vi "HDF5 Index.vi"(8 "error in (no error)":errorcluster, 11 "Mapping Type":enum16{"Dataset", "Variables"}(ring)=enum."Variables") -> (0 "error out":errorcluster, 3 "Mapping out":i32[](array[numeric]))   [LabVIEW 2011]
uses:
  User Interface VIs.lvlib
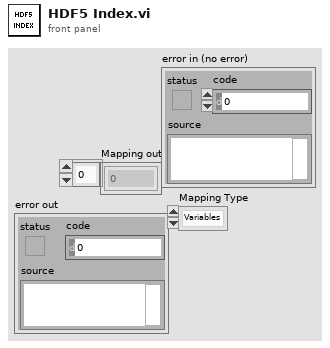
[diagram p1: front panel]
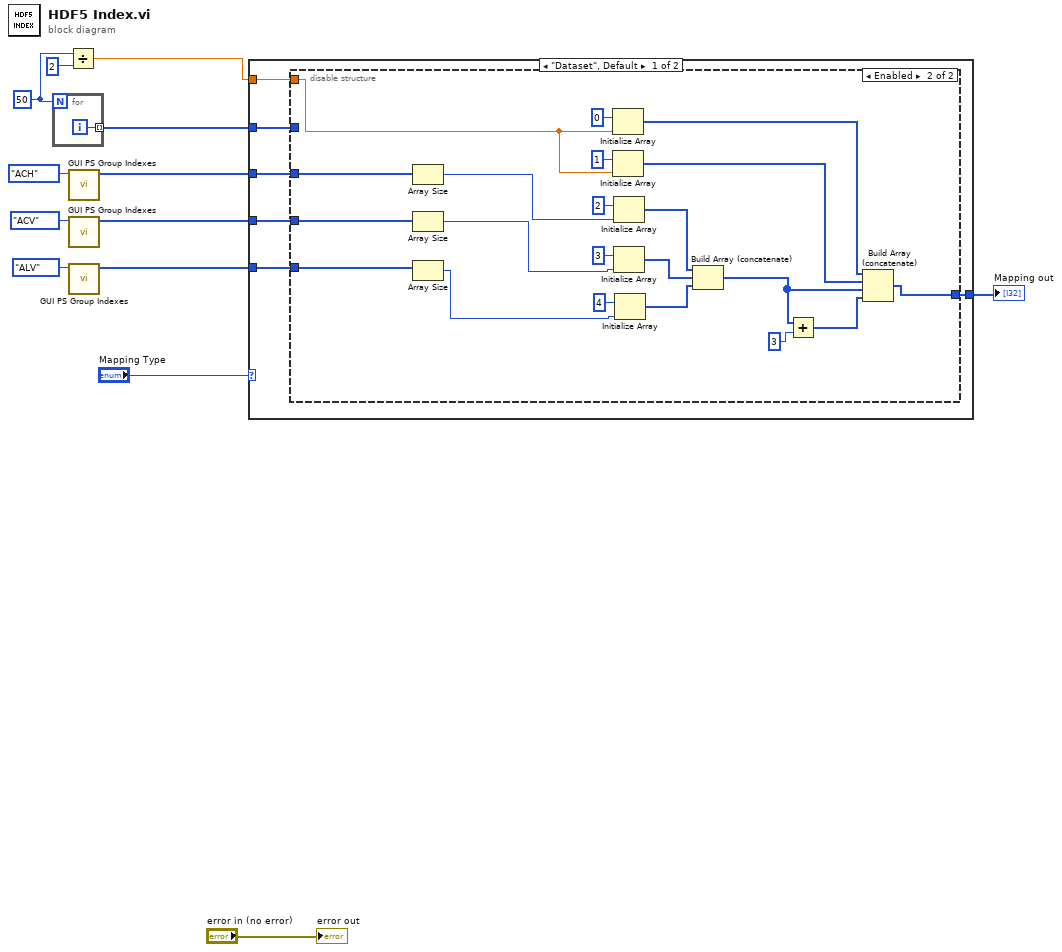
[diagram p0: block diagram]
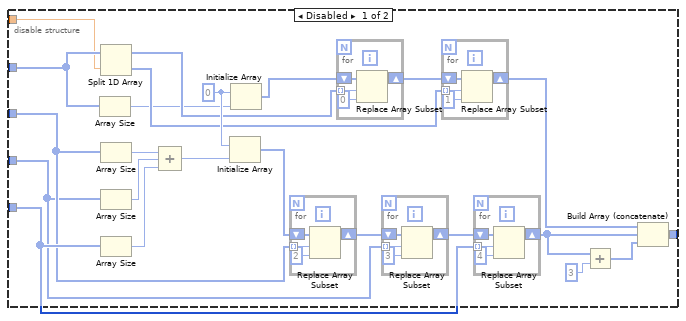
[diagram p2: hidden frame]
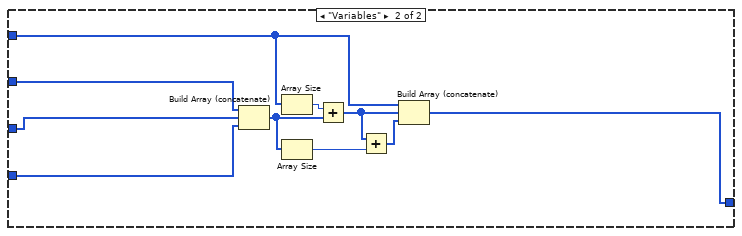
[diagram p3: hidden frame]
diagram:
  w7 = 50
  n1 = for {
    N: w7 -> [_]
    tunnel: [w14] -> w13 mode=indexing
    i -> [w14]
  }
  n2 = Divide(x=w7, y=2) -> (x/y=w9:dbl)
  n3 = call "GUI PS Group Indexes.vi"("PS Group"=enum16{"ACH", "ACV", "ALV"}."ACH") -> ("Indexes"=w10:i32[])  [unwired: 10 in]
  n4 = call "GUI PS Group Indexes.vi"("PS Group"=enum16{"ACH", "ACV", "ALV"}."ACV") -> ("Indexes"=w11:i32[])  [unwired: 10 in]
  n5 = call "GUI PS Group Indexes.vi"("PS Group"=enum16{"ACH", "ACV", "ALV"}."ALV") -> ("Indexes"=w12:i32[])  [unwired: 10 in]
  n6 = case shown="\"Dataset\", Default" "Mapping Type" {
    tunnel: w13 -> [w20 w89]
    tunnel: w12 -> [w19 w86]
    tunnel: w11 -> [w15 w87]
    tunnel: w10 -> [w18 w88]
    tunnel: w9 -> [w17 _]
    tunnel: [w16 w85] -> w2
    frame "Dataset", Default {
      n7 = disable-structure shown="Enabled" {
        disable-tunnel: w20 -> [w42 _]
        disable-tunnel: w19 -> [w41 w70]
        disable-tunnel: w18 -> [w40 w75]
        disable-tunnel: w17 -> [w37 w77]
        disable-tunnel: [w22 w64] -> w16
        disable-tunnel: w15 -> [w21 w71]
        frame Disabled {
          w43 = 0 ("size(s)")
          n8 = Array Size(array=w42) -> (size(s)=w29:i32)
          n9 = Split 1D Array(array=w42, index=w37) -> (first subarray=w39:i32[], second subarray=w38:i32[])
          n10 = Array Size(array=w40) -> (size(s)=w23:i32)
          n11 = Array Size(array=w21) -> (size(s)=w24:i32)
          n12 = Array Size(array=w41) -> (size(s)=w25:i32)
          n13 = Compound Arithmetic op=ADD(w23, w24, w25) -> (w26:i32)
          n14 = Initialize Array(w43, w26) -> (w32:i32[])
          n15 = Initialize Array(w43, w29) -> (w30:i32[])
          n16 = for {
            tunnel: w40 -> [w62] mode=indexing
            shift-right: [w61] -> w27
            shift-left: w32 -> [w63]
            n17 = Replace Array Subset(array=w63, new element=2 ("new element/subarray"), index=w62) -> (w61:i32[])
          }
          n18 = for {
            tunnel: w39 -> [w50] mode=indexing
            shift-right: [w49] -> w31
            shift-left: w30 -> [w51]
            n19 = Replace Array Subset(array=w51, new element=0 ("new element/subarray"), index=w50) -> (w49:i32[])
          }
          n20 = for {
            tunnel: w21 -> [w58] mode=indexing
            shift-right: [w57] -> w28
            shift-left: w27 -> [w59]
            n21 = Replace Array Subset(array=w59, new element=3 ("new element/subarray"), index=w58) -> (w57:i32[])
          }
          n22 = for {
            tunnel: w38 -> [w44] mode=indexing
            shift-right: [w46] -> w33
            shift-left: w31 -> [w47]
            tunnel: [w44] -> _ mode=indexing
            n23 = Replace Array Subset(array=w47, new element=1 ("new element/subarray"), index=w44) -> (w46:i32[])
          }
          n24 = for {
            tunnel: w41 -> [w54] mode=indexing
            shift-right: [w53] -> w34
            shift-left: w28 -> [w55]
            n25 = Replace Array Subset(array=w55, new element=4 ("new element/subarray"), index=w54) -> (w53:i32[])
          }
          n26 = Add(x=w34, y=3 ("size(s)")) -> (x+y=w36:i32[])
          n27 = Build Array (concatenate)(w33, w34, w36) -> (w22:i32[])
        }
        frame Enabled {
          n28 = Array Size(array=w75) -> (size(s)=w74:i32)
          n29 = Array Size(array=w71) -> (size(s)=w73:i32)
          n30 = Array Size(array=w70) -> (size(s)=w72:i32)
          n31 = Initialize Array(0 ("element"), w77) -> (w80:i32[])
          n32 = Initialize Array(1 ("element"), w77) -> (w79:i32[])
          n33 = Initialize Array(2 ("element"), w74) -> (w83:i32[])
          n34 = Initialize Array(3 ("element"), w73) -> (w82:i32[])
          n35 = Initialize Array(4 ("element"), w72) -> (w81:i32[])
          n36 = Build Array (concatenate)(w83, w82, w81) -> (w65:i32[])
          n37 = Add(x=w65, y=3 ("size(s)")) -> (x+y=w66:i32[])
          n38 = Build Array (concatenate)(w80, w79, w65, w66) -> (w64:i32[])
        }
      }
    }
    frame "Variables" {
      n39 = Build Array (concatenate)(w88, w87, w86) -> (w93:i32[])
      n40 = Array Size(array=w89) -> (size(s)=w94:i32)
      n41 = Array Size(array=w93) -> (size(s)=w91:i32)
      n42 = Add(x=w94, y=w93) -> (x+y=w90:i32[])
      n43 = Add(x=w90, y=w91) -> (x+y=w92:i32[])
      n44 = Build Array (concatenate)(w89, w90, w92) -> (w85:i32[])
    }
  }
  "Mapping out" <- w2
  "error out" <- "error in (no error)"
